vi "GlobalVariable.vi"() -> ()   [LabVIEW 2020]
panel:
  out "ConfigPath":string
  out "TempFolder":string
  out "SeqPath":string
  out "TestStandPath":string
  out "HistoryTodayFilePath":path
  out "PauseFile":path
  out "Pause":bool
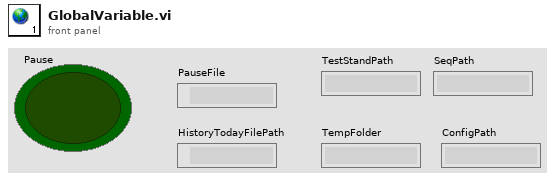
[diagram p1: front panel]
diagram:
